vi "3_ACK_NACK_Control_SubVI.vi"(11 "String":string) -> (2 "NACK":bool, 3 "ACK":bool)   [LabVIEW 2024]
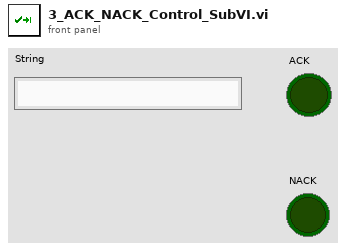
[diagram p1: front panel]
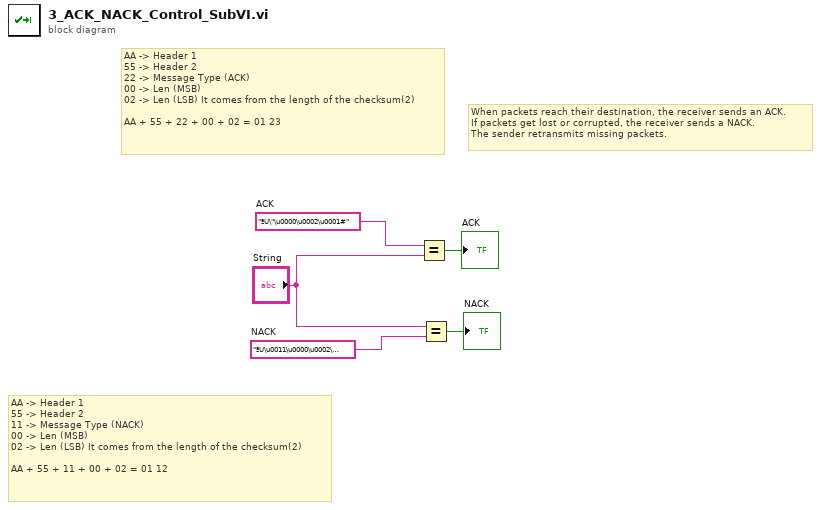
[diagram p0: block diagram]
diagram:
  w3 = "ªU\u0011\u0000\u0002\u0001\u0012"  # NACK
  w1 = "ªU\"\u0000\u0002\u0001#"  # ACK
  # "When packets reach their destination, the receiver sends an ACK.\nIf packets get lost or corrupted, the receiver sends a NACK.\nThe sender retransmits missing packets."
  # "AA -> Header 1\n55 -> Header 2\n11 -> Message Type (NACK)\n00 -> Len (MSB)\n02 -> Len (LSB) It comes from the length of the checksum(2)\n\nAA + 55 + 11 + 00 + 02 = 01 12"
  # "AA -> Header 1\n55 -> Header 2\n22 -> Message Type (ACK)\n00 -> Len (MSB)\n02 -> Len (LSB) It comes from the length of the checksum(2)\n\nAA + 55 + 22 + 00 + 02 = 01 23"
  n1 = Equal?(x=w1, y="String") -> (x = y?=→"ACK":bool)
  n2 = Equal?(x="String", y=w3) -> (x = y?=→"NACK":bool)
